vi "Add Artist.vi"(8 "error in (no error)":errorcluster, 10 "Artist Name":string, 11 "SQLite Connection in":refnum<class "Connection.lvclass">) -> (0 "error out":errorcluster, 3 "SQLite Connection out":refnum<class "Connection.lvclass">)   [LabVIEW 2015]
doc: "Adds a new artist to the database."
uses:
  <vilib>/drjdpowell/SQLite Library/SQL Connection/Connection.lvclass
  <vilib>/drjdpowell/SQLite Library/SQL Statement/SQL Statement.lvclass/SQL Statement.ctl
  <vilib>/drjdpowell/SQLite Library/SQL Statement/Bind Text.vi
  <vilib>/drjdpowell/SQLite Library/SQL Statement/Step.vi
  <vilib>/drjdpowell/SQLite Library/SQL Statement/Error Message.vi
  <vilib>/drjdpowell/SQLite Library/SQL Statement/SQL Statement.lvclass
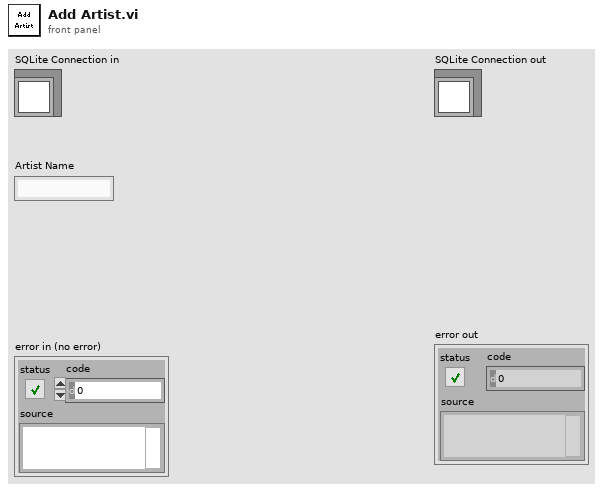
[diagram p1: front panel]
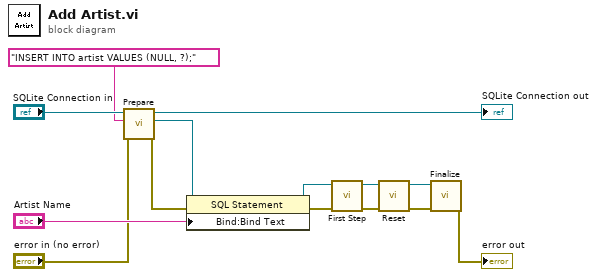
[diagram p0: block diagram]
diagram:
  n1 = call <vilib>:"Prepare.vi"("error in (no error)"="error in (no error)", "SQL"="INSERT INTO artist VALUES (NULL, ?);", "SQLite Connection in"="SQLite Connection in") -> ("error out"=w9:errorcluster, "SQL Statement"=w12:refnum<class "SQL Statement.lvclass">, "SQLite Connection"=→"SQLite Connection out":refnum<class "Connection.lvclass">)  [unwired: 4 in, 2 out]
  n2 = property class="SQL Statement"(reference=w12, error in=w9, "Bind:Bind Text"="Artist Name") -> (reference out=w8:refnum<class "SQL Statement.lvclass">, error out=w10:errorcluster)
  n3 = call <vilib>:"First Step.vi"("error in (no error)"=w10, "SQL Statement in"=w8) -> ("error out"=w6:errorcluster, "SQL Statement"=w7:refnum<class "SQL Statement.lvclass">)  [unwired: 7 in, 1 out]
  n4 = call <vilib>:"Reset.vi"("error in (no error)"=w6, "SQL Statement in"=w7) -> ("error out"=w4:errorcluster, "SQL Statement"=w5:refnum<class "SQL Statement.lvclass">)  [unwired: 8 in]
  n5 = call <vilib>:"Finalize.vi"("error in (no error)"=w4, "SQL Statement in"=w5) -> ("error out"=→"error out":errorcluster)  [unwired: 9 in]
